vi "Read Queue.vi"(11 "BluePlotHandle in":refnum<class "RocketPlotHandle.lvclass">) -> (1 "Valid?":bool, 2 "UE":refnum<user-event>, 3 "BluePlotHandle out":refnum<class "RocketPlotHandle.lvclass">)   [LabVIEW 2021, in "RocketPlotHandle.lvclass"]
uses:
  RocketPlotHandle.lvclass
  TypeDefs/plot handle queue data.ctl
  TypeDefs/Plot QSM action.ctl
  RocketPlotHandle.lvclass/RocketPlotHandle.ctl
  RocketPlot.lvlib
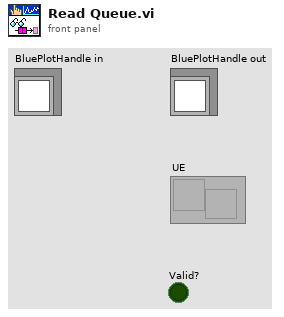
[diagram p1: front panel]
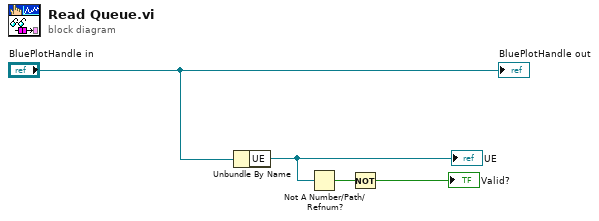
[diagram p0: block diagram]
diagram:
  n1 = Unbundle By Name("BluePlotHandle in") -> ("UE"=w1:refnum<user-event>)
  "UE" <- w1
  n2 = Not A Number/Path/Refnum?(number/path/refnum=w1) -> (NaN/Path/Refnum?=w4:bool)
  n3 = Not(x=w4) -> (.not. x?=→"Valid?":bool)
  "BluePlotHandle out" <- "BluePlotHandle in"
